vi "API_Stop Inspecting.vi"(8 "error in (no error)":errorcluster) -> (0 "error out":errorcluster)   [LabVIEW 2015, in "Tool Module.lvlib"]
doc: "Cancel the inspection in progress. This vi destroys the sample data notifier created by API_Start Inspecting.vi and used by API Get Sample Data.vi."
uses:
  Tool Module.lvlib
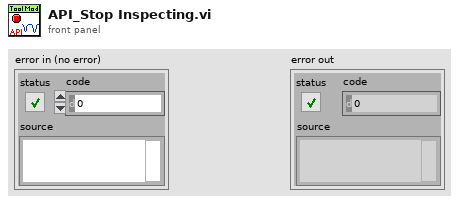
[diagram p1: front panel]
types:
  T1 = typedef "Tool Module.lvlib/_Sample Data Notifier--typedef.ctl" = refnum<notifier>
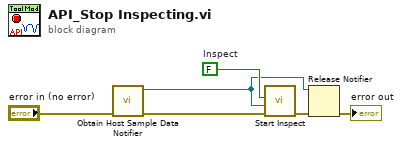
[diagram p0: block diagram]
diagram:
  w6 = FALSE  # Inspect
  n1 = call "Obtain Host Sample Data Notifier.vi"("error in (no error)"="error in (no error)") -> ("error out"=w3:errorcluster, "Sample Data Notifier"=w1:T1)  [unwired: 9 in]
  n2 = call "Start Inspect.vi"("error in (no error)"=w3, "Sample Data notifier"=w1, "Inspect"=w6) -> ("error out"=w2:errorcluster)  [unwired: 8 in]
  n3 = Release Notifier(notifier=w1, error in (no error)=w2) -> (error out=→"error out":errorcluster)  [unwired: 1 in, 2 out]
